vi "Dashboard Main.vi"() -> ()   [LabVIEW 2014]
uses:
  Autonomous Type.ctl
  <vilib>/event_ctls.llb/eventvkey.ctl
  <vilib>/Rock Robotics/WPI/Dashboard/WPI_DashboardLogging Global.vi
  <vilib>/Rock Robotics/Network Tables/SD Write Number.vi
  <vilib>/Rock Robotics/Network Tables/SD Read Number.vi
  <vilib>/Utility/config.llb/Write Key (String).vi
  <vilib>/Utility/config.llb/Write Key (I32).vi
  <vilib>/Utility/config.llb/NI_LVConfig.lvlib
panel:
  in  "TCP":refnum<k5>
  in  "Rec Mode":enum32{"Stop", "Record", "Playback"}(radio)
  in  "Vision":u16(ring) items=["Camera Off", "USB Camera SW", "USB Camera HW", "IP Camera"]
  out "Camera IP":string
  out "Image Message":string="Timeout in Camera Communications"
  in  "Dashboard Tab":T1(tab)
  out "Atonomous Type By Charlie":string
  in  "Camera Settings":T2={"Frame Rate"=30, "Compression"=30, "Size"=1} {"Frame Rate" scale=1.0..30.0; "Size" items=["640x480", "320x240", "160x120"]}
  out "MotorChart R":cluster{"Numeric":dbl, "Numeric":dbl}(graph)
  out "MotorChart L":T3(graph)
  out "MotorSliders R":cluster{"MotorSlide1":dbl, "MotorSlide2":dbl} {"MotorSlide2" scale=-1.0..1.0 scale format="%#_2e"; "MotorSlide1" scale=-1.0..1.0 scale format="%#_2e"}
  out "MotorSliders L":T4 {"MotorSlide4 2" scale=0.0..14.0 scale format="%#_2e"; "MotorSlide2" scale=-1.0..1.0 scale format="%#_2e"; "MotorSlide1" scale=-1.0..1.0 scale format="%#_2e"}
  out "Gyro":dbl(knob) scale=0.0..360.0
  out "JS1 Z":dbl(slide) scale=-1.0..1.0 scale format="%#_2e"
  out "JS1 Graph":cluster{"X":dbl, "Y":dbl}[](graph)
  out "JS1 Buttons":T5
  out "JS2 Z":dbl(slide) scale=-1.0..1.0 scale format="%#_2e"
  out "JS2 Graph":cluster{"X":dbl, "Y":dbl}[](graph)
  out "JS2 Buttons":T5
  out "Mode":T6(ring)=enum."Auto Disabled"
  in  "DB Camera Config":bool
  out "fps":dbl format="%#.1g"
  out "Mbps":dbl format="%#.1g"
  out "Mbps 2":bool
  in  "DB/String 9":string
  in  "DB/String 8":string
  in  "DB/String 7":string
  in  "DB/String 6":string
  in  "DB/String 5":string
  in  "DB/String 4":string
  in  "DB/String 3":string
  in  "DB/String 2":string
  in  "DB/String 1":string
  in  "DB/String 0":string
  in  "DB/Slider 0":dbl(slide) scale=0.0..5.0
  in  "DB/Slider 1":dbl(slide) scale=0.0..5.0
  in  "DB/Slider 2":dbl(slide) scale=0.0..5.0
  in  "DB/Slider 3":dbl(slide) scale=0.0..5.0
  out "DB/LED 3":bool
  out "DB/LED 2":bool
  out "DB/LED 1":bool
  out "DB/LED 0":bool
  in  "DB/Button 3":bool
  in  "DB/Button 2":bool
  in  "DB/Button 1":bool
  in  "DB/Button 0":bool caption="New Name"
  in  "Auto Type":T7
  in  "Test Slider":dbl(slide) scale=0.0..100.0 scale format="%#_3g"
  in  "On/Off":bool caption="Solenoid"
  in  "Test Name":u16(ring) items=["Select the test to run...", "Example Test", "-------------------------------", "List of tests is built in robot code.", "Replace with your own automated tests."]
  in  "Test Tree":string(tree)
  in  "Motor":cluster{"Value":dbl, "Enable":bool} {"Value" scale=-1.0..1.0 scale format="%#_3g"}
  out "Progress":T8 {"Test Progress" scale=0.0..100.0}
  in  "Rev/Fwd":cluster{"Forward":bool, "Reverse":bool}
  in  "Test Ring":u16(ring) items=["Monochrome", "Color"]
  in  "Listbox":i32(listbox)
  out "Tree":string(tree)
  out "Camera Image":T9(plugin-control)
  out "Boolean":bool
  # "Left"
  # "Front"
  # "Right"
  # "Battery"
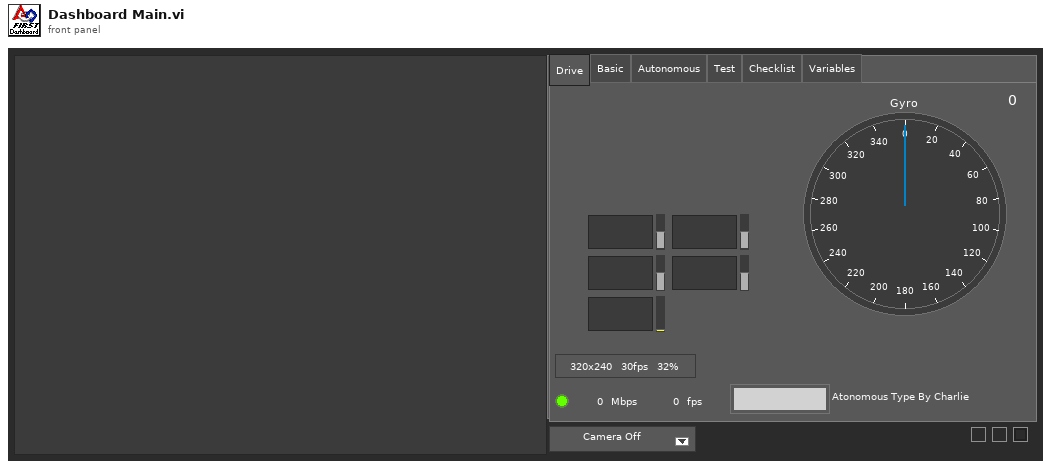
[diagram p1: front panel]
types:
  T1 = enum32{"Drive", "Basic", "Autonomous", "Test", "Checklist", "Variables"}
  T2 = cluster{"Frame Rate":i32, "Compression":i32, "Size":u16}
  T3 = cluster{"Numeric":dbl, "Numeric":dbl, "Battery V":dbl}
  T4 = cluster{"MotorSlide1":dbl, "MotorSlide2":dbl, "MotorSlide4 2":dbl}
  T5 = cluster{bool, bool, bool, bool, bool, bool, bool, bool, bool, bool, bool, bool}
  T6 = enum8{"Tele-Op Disabled", "Tele-Op Enabled", "Auto Disabled", "Auto Enabled", "Test Disabled", "Test Enabled", "Disconnected", "No Code", "E-Stop"}
  T7 = typedef "Autonomous Type.ctl" = enum16{"2 Totes + Turn", "Nothing", "3 Totes + Turn", "3 Totes + Strafe", "2 Totes + Strafe", "1 Tote", "Forward"}
  T8 = cluster{"Test Progress":u8, "Test Progress Text":string}
  T9 = typedef "IMAQ Image.ctl" = refnum<image>
  T10 = enum32{"Drive", "Basic", "Custom", "Test", "Checklist", "Variables"}
  T11 = typedef "Image Type" = u32
  T12 = cluster{"Camera Image":refnum<vi>, "Dashboard Tab":refnum<vi>, "Boolean":refnum<vi>, "Vision":refnum<vi>, "Rec Mode":refnum<vi>, "Test Slider":refnum<vi>, "On/Off ":refnum<vi>, "Test Ring":refnum<vi>, "Rev/Fwd":refnum<vi>, "Test Name":refnum<vi>, "Motor":refnum<vi>, "Progress":refnum<vi>, "CheckList":refnum<vi>, "Tree":refnum<vi>, "Test Tree":refnum<vi>}
  T13 = cluster{"Error Strings":string, "Disable Counts":cluster{u16, u16}, "Rail Faults":cluster{u16, u16, u16}, "Robot IP":string, "DB Mode":u8, "Event Info":cluster{"Name":string, "Type":u8, "Number":u16, "Replay":u8}, "Camera Addr":string}
  T14 = cluster{"Storage":cluster{"Disk Free":u64, "RAM Block":u32, "RAM free":u32}, "CPU Utilization":cluster{"CPU % ISR":sgl, "CPU % Time Crit":sgl, "CPU % Timed Str":sgl, "CPU % High":sgl, "CPU % Above":sgl, "CPU % Normal":sgl, "CPU % Low":sgl}, "CAN":cluster{"% Bus Utilization":sgl, "Bus Off Cnt":u32, "TX_FIFO Full Cnt":u32, "Receive Error Cnt":u8, "Transmit Error Cnt":u8}, "HID":cluster{"HID Outputs":u32, "Rumble Low":u16, "Rumble High":u16}[]}
  T15 = cluster{"Status bits":cluster{"Test Mode":bool, "Autonomous":bool, "Enabled":bool, "Code Start":bool, "Brownout":bool, "Reserved 2":bool, "Reserved 3":bool, "E-Stop":bool}, "Code Trace":cluster{"Disabled":bool, "TeleOp":bool, "Auto":bool, "Test":bool}, "Controller Type":enum16{"unknown", "cRIO", "roboRio"}, "Code?":enum16{"unknown", "noCode", "code"}, "Battery V":dbl}
  T16 = cluster{"Control Bits":cluster{"TestMode":bool, "Autonomous":bool, "Enabled":bool, "FMS Present":bool, bool, bool, bool, "E-Stop":bool}, "Team Station ":u8, "Countdown":sgl, "Joystick Values":cluster{"Axes":dbl[], "Buttons":bool[], "POVs":i16[]}[]}
  T17 = cluster{"Axes":dbl[], "Buttons":bool[], "POVs":i16[]}[]
  T18 = cluster{"Axes":dbl[], "Buttons":bool[], "POVs":i16[]}
  T19 = cluster{"Buttons[0]":bool, "Buttons[1]":bool, "Buttons[2]":bool, "Buttons[3]":bool, "Buttons[4]":bool, "Buttons[5]":bool, "Buttons[6]":bool, "Buttons[7]":bool, "Buttons[8]":bool, "Buttons[9]":bool, "Buttons[10]":bool, "Buttons[11]":bool}
  T20 = typedef "NI_LVConfig.lvlib/Config Data RefNum.ctl" = refnum<k1>
  T21 = cluster{"Operation":enum16{"Update", "Clear"}, "Color Box":u32}[]
  T22 = typedef "eventvkey.ctl" = enum16{"ASCII", "Enter", "Return", "Shift", "Ctrl", "Alt", "Cmd", "Opt", "Caps", "NumLock", "Clear", "Break", "Up", "Down", "Left", "Right", "Insert", "Delete", "Home", "End", "PageUp", "PageDown", "Escape", "Help", "Pause", "ScrollLock", "F1", "F2", "F3", "F4", "F5", "F6", "F7", "F8", "F9", "F10", "F11", "F12", "F13", "F14", "F15", "F16", "F17", "F18", "F19", "F20", "F21", "F22", "F23", "F24", "Play", "VolumeUp", "VolumeDown", "Mute", "Two Byte Char"}
  T23 = cluster{"Image Size":bool, "Image Type":bool, "Pixel Value":bool, "ROI Information":bool, "Zoom Factor":bool}
  T24 = enum8{"Enabled", "Disabled", "Disabled and Grayed Out"}
  T25 = cluster{"Operation":enum16{"Update", "Clear"}, "Color Box":u32}
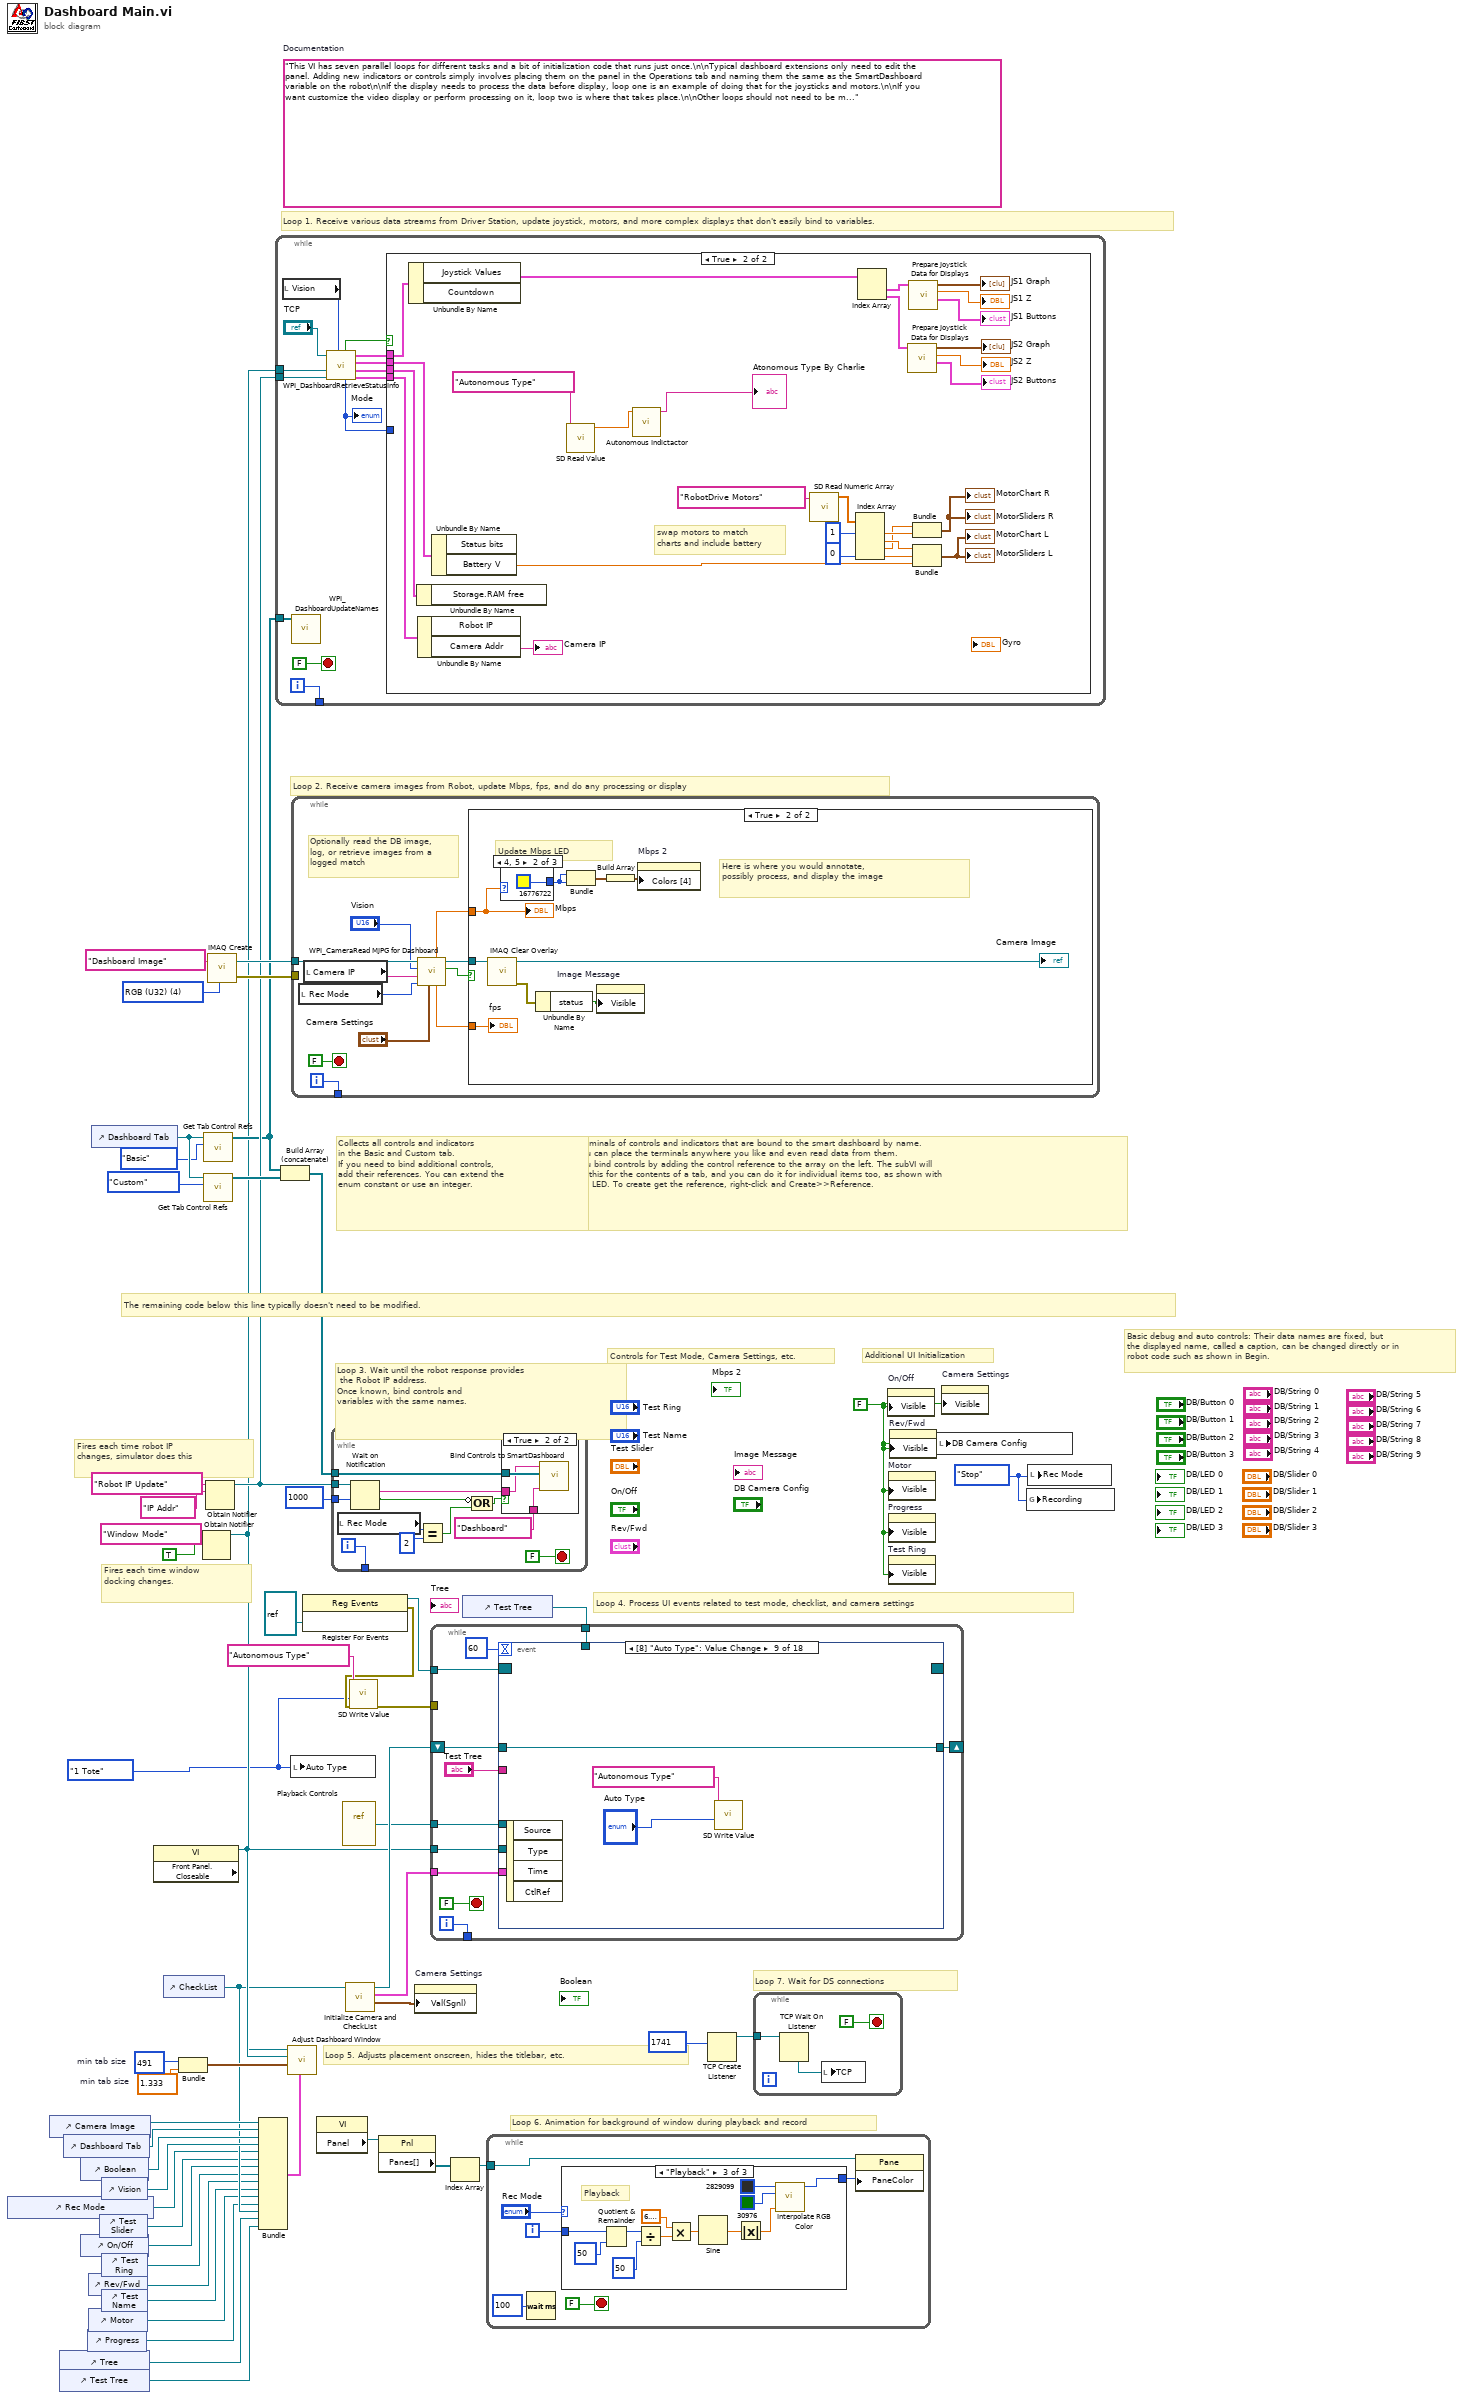
[diagram p0: block diagram]
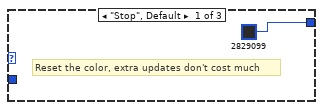
[diagram p3: hidden frame]
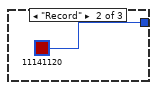
[diagram p4: hidden frame]
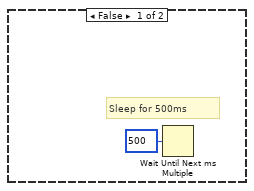
[diagram p6: hidden frame]
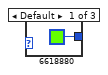
[diagram p7: hidden frame]
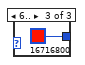
[diagram p8: hidden frame]
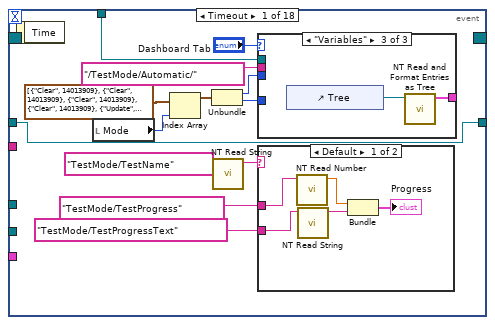
[diagram p9: hidden frame]
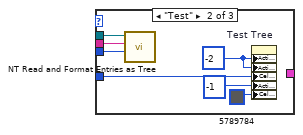
[diagram p11: hidden frame]
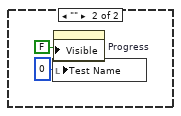
[diagram p12: hidden frame]
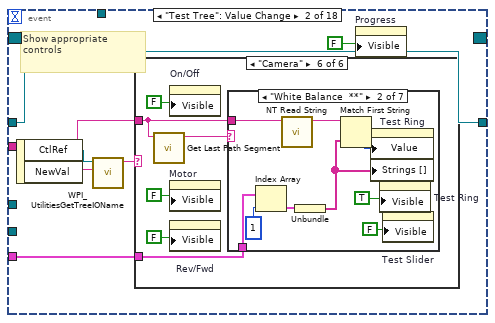
[diagram p13: hidden frame]
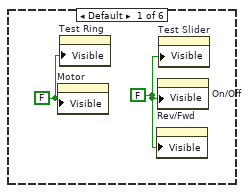
[diagram p14: hidden frame]
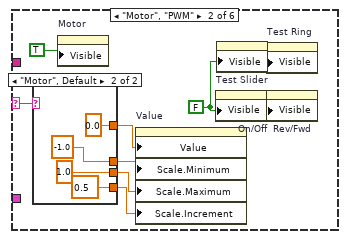
[diagram p15: hidden frame]
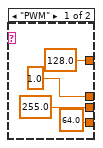
[diagram p16: hidden frame]
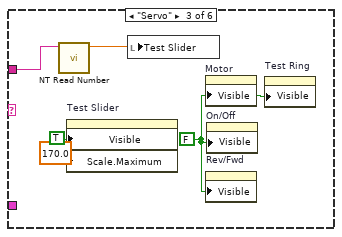
[diagram p17: hidden frame]
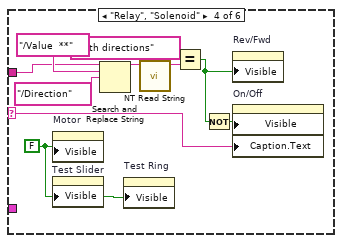
[diagram p18: hidden frame]
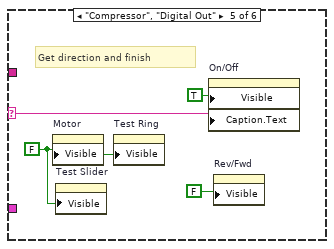
[diagram p19: hidden frame]
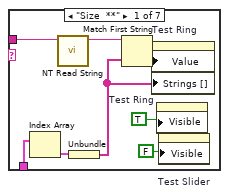
[diagram p20: hidden frame]
diagram:
  w1 = Autonomous_Type."1 Tote" ("Auto Type")
  w28 = 491  # min tab size
  w27 = 1.333  # min tab size
  w36 = enum32{"Stop", "Record", "Playback"}."Stop" ("Rec Mode")
  w10 = FALSE ("Visible")
  (unwired) "This VI has seven parallel loops for different tasks and a bit of initialization code that runs just once.\n\nTypical dashboard extensions only need to edit the panel. Adding new indicators or controls simply involves placing them on the panel in the Operations tab and naming them the same as the SmartDashboard variable on the robot\n\nIf the display needs to process the data before display, loop one is an example of doing that for the joysticks and motors.\n\nIf you want customize the video display or perform processing on it, loop two is where that takes place.\n\nOther loops should not need to be modified. They are pretty standard, and document the task they perform."  # Documentation
  w55 = T11 4 items=["Grayscale (U8)", "Grayscale (I16)", "Grayscale (SGL)", "Complex (CSG)", "RGB (U32)", "HSL (U32)", "RGB (U64)"] ("Image Type")
  # "Loop 7. Wait for DS connections"
  # "Basic debug and auto controls: Their data names are fixed, but\nthe displayed name, called a caption, can be changed directly or in\nrobot code such as shown in Begin."
  # "Controls for Test Mode, Camera Settings, etc."
  # "Additional UI Initialization"
  # "Loop 6. Animation for background of window during playback and record"
  # "Fires each time robot IP\nchanges, simulator does this"
  # "Fires each time window\ndocking changes."
  # "Collects all controls and indicators\nin the Basic and Custom tab.\nIf you need to bind additional controls,\nadd their references. You can extend the\nenum constant or use an integer."
  # "The remaining code below this line typically doesn't need to be modified."
  # "Loop 4. Process UI events related to test mode, checklist, and camera settings"
  # "Terminals of controls and indicators that are bound to the smart dashboard by name.\nYou can place the terminals anywhere you like and even read data from them.\nYou bind controls by adding the control reference to the array on the left. The subVI will\ndo this for the contents of a tab, and you can do it for individual items too, as shown with\nthe LED. To create get the reference, right-click and Create>>Reference."
  # "Loop 3. Wait until the robot response provides\n the Robot IP address.\nOnce known, bind controls and\nvariables with the same names."
  # "Loop 5. Adjusts placement onscreen, hides the titlebar, etc."
  # "Loop 1. Receive various data streams from Driver Station, update joystick, motors, and more complex displays that don't easily bind to variables."
  # "Loop 2. Receive camera images from Robot, update Mbps, fps, and do any processing or display"
  n1 = control-ref of="Rec Mode"() -> (w16:refnum<vi>)
  n2 = control-ref of="Camera Image"() -> (w31:refnum<vi>)
  n3 = control-ref of="Tree"() -> (w20:refnum<vi>)
  n4 = control-ref of="Test Tree"() -> (w19:refnum<vi>)
  n5 = control-ref of="Dashboard Tab"() -> (w30:refnum<vi>)
  n6 = control-ref of="Boolean"() -> (w25:refnum<vi>)
  n7 = control-ref of="On/Off"() -> (w14:refnum<vi>)
  n8 = control-ref of="Progress"() -> (w11:refnum<vi>)
  n9 = control-ref of="Rev/Fwd"() -> (w12:refnum<vi>)
  n10 = control-ref of="Motor"() -> (w17:refnum<vi>)
  n11 = control-ref of="Dashboard Tab"() -> (w34:refnum<vi>)
  n12 = control-ref of="Test Slider"() -> (w15:refnum<vi>)
  n13 = control-ref of="Vision"() -> (w29:refnum<vi>)
  n14 = control-ref of="Test Ring"() -> (w13:refnum<vi>)
  n15 = control-ref of="Test Name"() -> (w18:refnum<vi>)
  n16 = property class="VI" props=["Front Panel.Closeable"]() -> (reference out=w35:refnum<vi>)  [unwired: 2 in, 2 out]
  n17 = control-ref of="CheckList"() -> (w21:refnum<vi>)
  n18 = Bundle("min tab size"=w28, "min tab size"=w27) -> (w26:cluster{"min tab size":i32, "min tab size":dbl})  [unwired: 1 in]
  n19 = Obtain Notifier(name (unnamed)="Window Mode", notification data type=TRUE) -> (notifier out=w7:refnum<notifier>)  [unwired: 2 in, 2 out]
  n20 = call <vilib>:"Get Tab Control Refs.vi"("Page Index"=T10."Basic" ("Dashboard Tab"), "TabControl in"=w34) -> ("ControlsOnPage"=w8:refnum<vi>[])  [unwired: 9 in]
  n21 = call <vilib>:"Get Tab Control Refs.vi"("Page Index"=T10."Custom" ("Dashboard Tab"), "TabControl in"=w34) -> ("ControlsOnPage"=w33:refnum<vi>[])  [unwired: 9 in]
  n22 = Obtain Notifier(name (unnamed)="Robot IP Update", notification data type="IP Addr" ("name (unnamed)")) -> (notifier out=w9:refnum<notifier>)  [unwired: 2 in, 2 out]
  n23 = call "IMAQ Create"("Image Name"="Dashboard Image", "Image Type"=w55) -> ("New Image"=w53:T9, "error out"=w52:errorcluster)  [unwired: 2 in, 1 out]
  n24 = Bundle("Camera Image"=w31, "Dashboard Tab"=w30, "Boolean"=w25, "Vision"=w29, "Rec Mode"=w16, "Test Slider"=w15, "On/Off"=w14, "Test Ring"=w13, "Rev/Fwd"=w12, "Test Name"=w18, "Motor"=w17, "Progress"=w11, "CheckList"=w21, "Tree"=w20, "Test Tree"=w19) -> (w22:T12)  [unwired: 1 in]
  n25 = while {
    tunnel: [w67] -> _
    tunnel: w9 -> [w61]
    tunnel: w8 -> [w60]
    tunnel: w7 -> [w56]
    i -> [w67]
    stop <- FALSE stop-if-true
    n26 = local read "Vision"() -> (w58:u16)
    n27 = call <vilib>:"WPI_DashboardUpdateNames.vi"("Controls on Tab"=w60) -> ()  [unwired: 11 in]
    n28 = call <vilib>:"WPI_DashboardRetrieveStatusInfo.vi"("Vision"=w58, "Binding Refnum"=w61, "Window Mode Notifier"=w56, "TCP Cnx"="TCP") -> ("Power and Errors"=w62:T13, "Robot Metrics"=w65:T14, "Status Info"=w66:T15, "Control Info"=w63:T16, "Robot Mode"=w59:T6, "Process?"=w64:bool)  [unwired: 2 in]
    "Mode" <- w59
    n29 = case shown="True" w64 {
      tunnel: w66 -> [_ w96]
      tunnel: w65 -> [_ w95]
      tunnel: w63 -> [_ w94]
      tunnel: w62 -> [_ w93]
      tunnel: w59 -> [_ _]
      frame False {
      }
      frame True {
        # "swap motors to match\ncharts and include battery"
        n30 = Unbundle By Name(w94) -> ("Joystick Values"=w81:T17)  [unwired: 1 out]
        n31 = Unbundle By Name(w95) -> ()  [unwired: 1 out]
        n32 = Unbundle By Name(w93) -> ("Camera Addr"=→"Camera IP":string)  [unwired: 1 out]
        n33 = Unbundle By Name(w96) -> ("Battery V"=w82:dbl)  [unwired: 1 out]
        n34 = call-poly <vilib>:"SD Read Value.vi"("Name"="Autonomous Type") -> ("Numeric"=w70:dbl)  [unwired: 8 in, 2 out]
        n35 = call "Autonomous Indictactor.vi"("Int In"=w70) -> ("String Out"=→"Atonomous Type By Charlie":string)  [unwired: 10 in]
        n36 = call <vilib>:"SD Read Numeric Array.vi"("Name"="RobotDrive Motors") -> ("Numeric Array"=w84:dbl[])  [unwired: 8 in, 2 out]
        n37 = Index Array(array=w84, index #1=1, index #4=0) -> (element #1=w88:dbl, element #2=w89:dbl, element #3=w87:dbl, element #4=w92:dbl)  [unwired: 2 in]
        n38 = Index Array(array=w81) -> (element #1=w80:T18, element #2=w75:T18)  [unwired: 2 in]
        n39 = call "Prepare Joystick Data for Displays.vi"("Joystick Values"=w75) -> ("Buttons"=→"JS2 Buttons":T19, "Z Axis"=→"JS2 Z":dbl, "Cartesian Data"=→"JS2 Graph":cluster{"X axis":dbl, "X axis":dbl}[])  [unwired: 8 in]
        n40 = call "Prepare Joystick Data for Displays.vi"("Joystick Values"=w80) -> ("Buttons"=→"JS1 Buttons":T19, "Z Axis"=→"JS1 Z":dbl, "Cartesian Data"=→"JS1 Graph":cluster{"X axis":dbl, "X axis":dbl}[])  [unwired: 8 in]
        n41 = Bundle("Numeric"=w87, "Numeric"=w88) -> (→"MotorChart R" →"MotorSliders R":cluster{"Numeric":dbl, "Numeric":dbl})  [unwired: 1 in]
        n42 = Bundle("Numeric"=w89, "Numeric"=w92, "Battery V"=w82) -> (→"MotorChart L" →"MotorSliders L":T3)  [unwired: 1 in]
      }
    }
  }
  n43 = Build Array (concatenate)(w8, w33) -> (w32:refnum<vi>[])
  n44 = call "Adjust Dashboard Window.vi"("Sizing Refnums"=w22, "Size Constraints"=w26, "VI"=w35, "Notifier in"=w7) -> ()  [unwired: 8 in]
  n45 = local write "Auto Type"(w1) -> ()
  n46 = while {
    tunnel: w53 -> [w105]
    tunnel: w52 -> [_]
    tunnel: [w106] -> _
    i -> [w106]
    stop <- FALSE stop-if-true
    # "Optionally read the DB image,\nlog, or retrieve images from a\nlogged match"
    n47 = local read "Rec Mode"() -> (w99:enum32{"Stop", "Record", "Playback"})
    n48 = local read "Camera IP"() -> (w97:string)
    n49 = call <vilib>:"WPI_CameraRead MJPG for Dashboard.vi"("Camera Settings"="Camera Settings", "Rec Mode"=w99, "Camera IP"=w97, "Camera Mode"="Vision", "Refnum in"=w105) -> ("Active"=w103:bool, "Refnum out"=w104:T9, "FPS"=w102:dbl, "Bandwidth (Mbps)"=w101:dbl)  [unwired: 3 in]
    n50 = case shown="True" w103 {
      tunnel: w104 -> [_ w112]
      tunnel: w101 -> [_ w111]
      tunnel: w102 -> [_ w109]
      frame False {
        # "Sleep for 500ms"
        n51 = Wait Until Next ms Multiple(millisecond multiple=u32 500) -> ()  [unwired: 1 out]
      }
      frame True {
        # "Here is where you would annotate,\npossibly process, and display the image"
        # "Update Mbps LED"
        n52 = call "IMAQ Clear Overlay"("Image"=w112) -> ("error out"=w116:errorcluster, "Image Out"=→"Camera Image":T9)  [unwired: 2 in, 7 out]
        n53 = case shown="4, 5" w111 {
          tunnel: [u32 6618880 ("Color Box") u32 16776722 ("Color Box") u32 16716800 ("Color Box")] -> w113
          frame Default {
          }
          frame 4, 5 {
          }
          frame 6.. {
          }
        }
        n54 = Unbundle By Name(w116) -> ("status"=w117:bool)
        n55 = Bundle("Color Box"=w113, "Color Box"=w113) -> (w115:cluster{"Color Box":u32, "Color Box":u32})  [unwired: 1 out]
        n56 = property on="Image Message" class="Str"("Visible"=w117) -> ()  [unwired: 2 in, 2 out]
        n57 = Build Array(w115) -> (w114:cluster{"Color Box":u32, "Color Box":u32}[])
        n58 = property on="Mbps 2" class="Bool (strict)"("Colors [4]"=w114) -> ()  [unwired: 2 in, 2 out]
        "Mbps" <- w111
        "fps" <- w109
      }
    }
  }
  n59 = register-events(refnum<vi> refnum) -> (reference out=w39:refnum<event-registration>, error out=w3:errorcluster)  [unwired: 2 in]
  n60 = property class="VI"() -> ("Panel"=w42:refnum<vi>)  [unwired: 2 in, 2 out]
  n61 = while {
    tunnel: w32 -> [w132]
    tunnel: w9 -> [w130]
    tunnel: [w128] -> _
    tunnel: u32 1000 ("milliseconds to wait") -> [w127]
    i -> [w128]
    stop <- FALSE stop-if-true
    n62 = local read "Rec Mode"() -> (w123:enum32{"Stop", "Record", "Playback"})
    n63 = Wait on Notification(notifier=w130, timeout in ms (-1)=w127) -> (notification=w129:string, timed out?=w125:bool)  [unwired: 2 in, 2 out]
    n64 = Equal?(x=w123, y=u16 2 ("Rec Mode")) -> (x = y?=w124:bool)
    n65 = Compound Arithmetic op=OR(invert w125, w124) -> (w126:bool)
    n66 = case shown="True" w126 {
      tunnel: w132 -> [_ w135]
      tunnel: w129 -> [_ w134]
      tunnel: "Dashboard" -> [_ w133]
      frame False {
      }
      frame True {
        n67 = call <vilib>:"Bind Controls to SmartDashboard.vi"("Client Name"=w133, "Bound Control Refs"=w135, "Server IP Address"=w134) -> ()  [unwired: 9 in]
      }
    }
  }
  n68 = vi-ref "Playback Controls.vi"() -> (w40:refnum<vi>)
  n69 = call "Initialize Camera and CheckList.vi"("ListBox in"=w21) -> ("Cluster"=w46:cluster{"value":i32, "value":i32, "index":i32}, "Array"=w47:cluster{string[]}[], "File Refnum"=w45:T20)  [unwired: 8 in]
  n70 = call-poly <vilib>:"SD Write Value.vi"("error in"=w3, "Numeric"=w1, "Name"="Autonomous Type") -> ("error out"=w2:errorcluster)  [unwired: 7 in, 1 out]
  n71 = property class="Pnl"(reference=w42) -> ("Panes[]"=w43:refnum<vi>[])  [unwired: 1 in, 2 out]
  n72 = property on="Camera Settings" class="Clust (strict)"("Val(Sgnl)"=w46) -> ()  [unwired: 2 in, 2 out]
  n73 = Index Array(array=w43) -> (element=w41:refnum<vi>)  [unwired: 1 in]
  n74 = control-ref of="Test Tree"() -> (w44:refnum<vi>)
  n75 = while {
    tunnel: w47 -> [w143]
    shift-right: [w142] -> _
    shift-left: w45 -> [w141]
    tunnel: [w140] -> _
    tunnel: w44 -> [w139]
    tunnel: w40 -> [w138]
    tunnel: w39 -> [w137]
    tunnel: w35 -> [w136]
    tunnel: w2 -> [_]
    i -> [w140]
    stop <- FALSE stop-if-true
    n76 = event shown="[8] \"Auto Type\": Value Change" {
      selector: w137 -> [_ _ _ _ _ _ _ _ _ _ _ _ _ _ _ _ _ _]
      dyn-events: [_ _ _ _ _ _ _ _ _ _ _ _ _ _ w384 _ _ _] -> _
      timeout: u32 60 ("milliseconds to wait") -> [_ _ _ _ _ _ _ _ _ _ _ _ _ _ _ _ _ _]
      tunnel: w139 -> [w155 _ _ _ _ _ _ _ _ _ _ _ _ _ _ _ _ _]
      tunnel: "Test Tree" -> [_ _ _ _ _ _ _ _ _ w353 w361 w363 w367 w375 _ _ _ _]
      tunnel: w143 -> [_ w177 _ _ _ _ w314 w344 _ _ _ _ _ _ _ _ _ _]
      tunnel: [w151 w176 w275 w280 w288 w300 w313 w337 w351 w352 w359 w362 w366 w374 w386 w400 w401 w411] -> w142
      tunnel: w141 -> [w151 w176 w275 w280 w288 w300 w312 w337 w351 w352 w359 w362 w366 w374 w386 w400 w401 w411]
      tunnel: w138 -> [_ _ _ _ _ _ _ _ _ _ _ _ _ _ w387 _ w404 _]
      tunnel: w136 -> [_ _ _ _ _ _ _ _ _ _ _ _ _ _ w382 _ _ _]
      event Timeout {
        n77 = event-data() -> ()  [unwired: 1 in, 1 out]
        n78 = local read "Mode"() -> (w154:T6)
        n79 = Index Array(array=T21 [{"Operation"=enum."Clear", "Color Box"=14013909}, {"Operation"=enum."Clear", "Color Box"=14013909}, {"Operation"=enum."Clear", "Color Box"=14013909}, {"Operation"=enum."Clear", "Color Box"=14013909}, {"Operation"=enum."Update", "Color Box"=14013909}, {"Operation"=enum."Update", "Color Box"=16777215}, {"Operation"=enum."Clear", "Color Box"=14013909}, {"Operation"=enum."Clear", "Color Box"=14013909}, {"Operation"=enum."Clear", "Color Box"=14013909}], index=w154) -> (element=w149:T25)
        n80 = Unbundle(w149) -> ("Operation"=w148:enum16{"Update", "Clear"}, "Color Box"=w147:u32)
        n81 = call <vilib>:"NT Read String.vi"("Name"="TestMode/TestName") -> ("String"=w158:string)  [unwired: 9 in, 1 out]
        n82 = case shown="\"Variables\"" "Dashboard Tab" {
          tunnel: w155 -> [_ w166 _]
          tunnel: "/TestMode/Automatic/" ("Name Pattern") -> [_ w165 _]
          tunnel: w148 -> [_ w164 _]
          tunnel: [_ _ w168] -> _
          tunnel: w147 -> [_ w160 _]
          frame "Autonomous", Default {
          }
          frame "Test" {
            w163 = -2 ("Active Item:Row Number")
            n83 = call <vilib>:"NT Read and Format Entries as Tree.vi"("Operation"=w164, "Name Pattern"=w165, "Tree Refnum"=w166) -> ()  [unwired: 7 in, 2 out]
            n84 = property on="Test Tree" class="Tree (strict)"("Active Item Row Number"=w163, "ActiveColNum"=w163, "CellBG"=w160, "Active Item Row Number"=-1 ("Active Item:Row Number"), "CellBG"=u32 5789784 ("Color Box")) -> ()  [unwired: 2 in, 2 out]
          }
          frame "Variables" {
            n85 = control-ref of="Tree"() -> (w167:refnum<vi>)
            n86 = call <vilib>:"NT Read and Format Entries as Tree.vi"("Tree Refnum"=w167) -> ("Formatted Strings"=w168:cluster{"Name":string, "Value":string}[])  [unwired: 9 in, 1 out]
          }
        }
        n87 = case shown="Default" w158 {
          tunnel: "TestMode/TestProgress" ("Name") -> [w170 _]
          tunnel: "TestMode/TestProgressText" ("Name") -> [w169 _]
          frame Default {
            n88 = call <vilib>:"NT Read Number.vi"("Name"=w170) -> ("Numeric"=w171:dbl)  [unwired: 9 in, 1 out]
            n89 = call <vilib>:"NT Read String.vi"("Name"=w169) -> ("String"=w172:string)  [unwired: 9 in, 1 out]
            n90 = Bundle("Numeric"=w171, "String"=w172) -> (→"Progress":cluster{"Numeric":dbl, "String":string})  [unwired: 1 in]
          }
          frame "" {
            n91 = local write "Test Name"(u16 0) -> ()
            n92 = property on="Progress" class="Clust (strict)"("Visible"=FALSE) -> ()  [unwired: 2 in, 2 out]
          }
        }
      }
      event "Test Tree": Value Change {
        # "Show appropriate\ncontrols"
        n93 = event-data() -> ("CtlRef"=w180:refnum<vi>, "NewVal"=w178:string)  [unwired: 1 in]
        n94 = call <vilib>:"WPI_UtilitiesGetTreeIOName.vi"("NewVal"=w178, "TreeControl in"=w180) -> ("I/O Name"=w181:string)  [unwired: 9 in]
        n95 = case shown="\"Camera\"" w181 {
          selector: w181 -> [_ w188 _ w206 w215 _]
          tunnel: w178 -> [_ _ w203 w205 _ w222]
          tunnel: w177 -> [_ _ _ _ _ w221]
          frame Default {
            w183 = FALSE ("Visible")
            w182 = FALSE ("Visible")
            n96 = property on="Motor" class="Clust (strict)"("Visible"=w182) -> ()  [unwired: 2 in, 2 out]
            n97 = property on="Test Ring" class="Ring (strict)"("Visible"=w182) -> ()  [unwired: 2 in, 2 out]
            n98 = property on="Rev/Fwd" class="Clust (strict)"("Visible"=w183) -> ()  [unwired: 2 in, 2 out]
            n99 = property on="On/Off" class="Bool (strict)"("Visible"=w183) -> ()  [unwired: 2 in, 2 out]
            n100 = property on="Test Slider" class="Slide (strict)"("Visible"=w183) -> ()  [unwired: 2 in, 2 out]
          }
          frame "Motor", "PWM" {
            w189 = FALSE ("Visible")
            n101 = case shown="\"Motor\", Default" w188 {
              tunnel: [1.0 ("Value") -1.0 ("Value")] -> w187
              tunnel: [255.0 ("Value") 1.0 ("Value")] -> w186
              tunnel: [128.0 ("Value") 0.0 ("Value")] -> w185
              tunnel: [64.0 ("Value") 0.5 ("Value")] -> w184
              frame "PWM" {
              }
              frame "Motor", Default {
              }
            }
            n102 = property on="Motor" class="Clust (strict)"("Visible"=TRUE) -> ()  [unwired: 2 in, 2 out]
            n103 = property on="Value" class="Slide (strict)"("Value"=w185, "Scale.Minimum"=w187, "Scale.Maximum"=w186, "Scale.Increment"=w184) -> ()  [unwired: 2 in, 2 out]
            n104 = property on="On/Off" class="Bool (strict)"("Visible"=w189) -> ()  [unwired: 2 in, 2 out]
            n105 = property on="Test Slider" class="Slide (strict)"("Visible"=w189) -> ()  [unwired: 2 in, 2 out]
            n106 = property on="Test Ring" class="Ring (strict)"("Visible"=w189) -> ()  [unwired: 2 in, 2 out]
            n107 = property on="Rev/Fwd" class="Clust (strict)"("Visible"=w189) -> ()  [unwired: 2 in, 2 out]
          }
          frame "Servo" {
            w201 = FALSE ("Visible")
            n108 = call <vilib>:"NT Read Number.vi"("Name"=w203) -> ("Numeric"=w202:dbl)  [unwired: 9 in, 1 out]
            n109 = property on="Test Slider" class="Slide (strict)"("Visible"=TRUE, "Scale.Maximum"=170.0 ("Scale.Range:Maximum")) -> ()  [unwired: 2 in, 2 out]
            n110 = local write "Test Slider"(w202) -> ()
            n111 = property on="Motor" class="Clust (strict)"("Visible"=w201) -> ()  [unwired: 2 in, 2 out]
            n112 = property on="Rev/Fwd" class="Clust (strict)"("Visible"=w201) -> ()  [unwired: 2 in, 2 out]
            n113 = property on="On/Off" class="Bool (strict)"("Visible"=w201) -> ()  [unwired: 2 in, 2 out]
            n114 = property on="Test Ring" class="Ring (strict)"("Visible"=w201) -> ()  [unwired: 2 in, 2 out]
          }
          frame "Relay", "Solenoid" {
            w204 = FALSE ("Visible")
            n115 = property on="Motor" class="Clust (strict)"("Visible"=w204) -> ()  [unwired: 2 in, 2 out]
            n116 = property on="Test Slider" class="Slide (strict)"("Visible"=w204) -> ()  [unwired: 2 in, 2 out]
            n117 = Search and Replace String(input string=w205, search string="/Value  **", replace string="/Direction") -> (result string=w211:string)  [unwired: 5 in, 3 out]
            n118 = property on="Test Ring" class="Ring (strict)"("Visible"=w204) -> ()  [unwired: 2 in, 2 out]
            n119 = call <vilib>:"NT Read String.vi"("Name"=w211) -> ("String"=w209:string)  [unwired: 9 in, 1 out]
            n120 = Equal?(x="Both directions", y=w209) -> (x = y?=w207:bool)
            n121 = Not(x=w207) -> (.not. x?=w208:bool)
            n122 = property on="Rev/Fwd" class="Clust (strict)"("Visible"=w207) -> ()  [unwired: 2 in, 2 out]
            n123 = property on="On/Off" class="Bool (strict)"("Visible"=w208, "Caption.Text"=w206) -> ()  [unwired: 2 in, 2 out]
          }
          frame "Compressor", "Digital Out" {
            w214 = FALSE ("Visible")
            # "Get direction and finish"
            n124 = property on="Motor" class="Clust (strict)"("Visible"=w214) -> ()  [unwired: 2 in, 2 out]
            n125 = property on="Test Slider" class="Slide (strict)"("Visible"=w214) -> ()  [unwired: 2 in, 2 out]
            n126 = property on="Test Ring" class="Ring (strict)"("Visible"=w214) -> ()  [unwired: 2 in, 2 out]
            n127 = property on="On/Off" class="Bool (strict)"("Visible"=TRUE, "Caption.Text"=w215) -> ()  [unwired: 2 in, 2 out]
            n128 = property on="Rev/Fwd" class="Clust (strict)"("Visible"=FALSE) -> ()  [unwired: 2 in, 2 out]
          }
          frame "Camera" {
            n129 = call <vilib>:"Get Last Path Segment.vi"("String in"=w222) -> ("String out"=w223:string)  [unwired: 10 in]
            n130 = property on="On/Off" class="Bool (strict)"("Visible"=FALSE) -> ()  [unwired: 2 in, 2 out]
            n131 = property on="Motor" class="Clust (strict)"("Visible"=FALSE) -> ()  [unwired: 2 in, 2 out]
            n132 = property on="Rev/Fwd" class="Clust (strict)"("Visible"=FALSE) -> ()  [unwired: 2 in, 2 out]
            n133 = case shown="\"White Balance  **\"" w223 {
              tunnel: w222 -> [w229 w238 w247 w256 w265 _ w271]
              tunnel: w221 -> [w227 w235 w244 w253 w262 _ _]
              frame "Size  **" {
                n134 = Index Array(array=w227) -> (element=w226:cluster{string[]})  [unwired: 1 in]
                n135 = call <vilib>:"NT Read String.vi"("Name"=w229) -> ("String"=w228:string)  [unwired: 9 in, 1 out]
                n136 = Unbundle(w226) -> (w224:string[])
                n137 = Match First String(2:w224, 3:w228) -> (0:w225:i32)  [unwired: 1 out]
                n138 = property on="Test Ring" class="Ring (strict)"("Value"=w225, "Strings []"=w224) -> ()  [unwired: 2 in, 2 out]
                n139 = property on="Test Ring" class="Ring (strict)"("Visible"=TRUE) -> ()  [unwired: 2 in, 2 out]
                n140 = property on="Test Slider" class="Slide (strict)"("Visible"=FALSE) -> ()  [unwired: 2 in, 2 out]
              }
              frame "White Balance  **" {
                n141 = Index Array(array=w235, index=1) -> (element=w236:cluster{string[]})
                n142 = call <vilib>:"NT Read String.vi"("Name"=w238) -> ("String"=w237:string)  [unwired: 9 in, 1 out]
                n143 = Unbundle(w236) -> (w233:string[])
                n144 = Match First String(2:w233, 3:w237) -> (0:w232:i32)  [unwired: 1 out]
                n145 = property on="Test Ring" class="Ring (strict)"("Value"=w232, "Strings []"=w233) -> ()  [unwired: 2 in, 2 out]
                n146 = property on="Test Ring" class="Ring (strict)"("Visible"=TRUE) -> ()  [unwired: 2 in, 2 out]
                n147 = property on="Test Slider" class="Slide (strict)"("Visible"=FALSE) -> ()  [unwired: 2 in, 2 out]
              }
              frame "Exposure  **" {
                n148 = Index Array(array=w244, index=2) -> (element=w245:cluster{string[]})
                n149 = call <vilib>:"NT Read String.vi"("Name"=w247) -> ("String"=w246:string)  [unwired: 9 in, 1 out]
                n150 = Unbundle(w245) -> (w241:string[])
                n151 = Match First String(2:w241, 3:w246) -> (0:w242:i32)  [unwired: 1 out]
                n152 = property on="Test Ring" class="Ring (strict)"("Value"=w242, "Strings []"=w241) -> ()  [unwired: 2 in, 2 out]
                n153 = property on="Test Ring" class="Ring (strict)"("Visible"=TRUE) -> ()  [unwired: 2 in, 2 out]
                n154 = property on="Test Slider" class="Slide (strict)"("Visible"=FALSE) -> ()  [unwired: 2 in, 2 out]
              }
              frame "Exposure Priority  **" {
                n155 = Index Array(array=w253, index=3) -> (element=w254:cluster{string[]})
                n156 = call <vilib>:"NT Read String.vi"("Name"=w256) -> ("String"=w255:string)  [unwired: 9 in, 1 out]
                n157 = Unbundle(w254) -> (w250:string[])
                n158 = Match First String(2:w250, 3:w255) -> (0:w251:i32)  [unwired: 1 out]
                n159 = property on="Test Ring" class="Ring (strict)"("Value"=w251, "Strings []"=w250) -> ()  [unwired: 2 in, 2 out]
                n160 = property on="Test Ring" class="Ring (strict)"("Visible"=TRUE) -> ()  [unwired: 2 in, 2 out]
                n161 = property on="Test Slider" class="Slide (strict)"("Visible"=FALSE) -> ()  [unwired: 2 in, 2 out]
              }
              frame "Color Enable  **" {
                n162 = Index Array(array=w262, index=4) -> (element=w263:cluster{string[]})
                n163 = call <vilib>:"NT Read String.vi"("Name"=w265) -> ("String"=w264:string)  [unwired: 9 in, 1 out]
                n164 = Unbundle(w263) -> (w259:string[])
                n165 = Match First String(2:w259, 3:w264) -> (0:w260:i32)  [unwired: 1 out]
                n166 = property on="Test Ring" class="Ring (strict)"("Value"=w260, "Strings []"=w259) -> ()  [unwired: 2 in, 2 out]
                n167 = property on="Test Ring" class="Ring (strict)"("Visible"=TRUE) -> ()  [unwired: 2 in, 2 out]
                n168 = property on="Test Slider" class="Slide (strict)"("Visible"=FALSE) -> ()  [unwired: 2 in, 2 out]
              }
              frame Default {
                n169 = property on="Test Ring" class="Ring (strict)"("Visible"=FALSE) -> ()  [unwired: 2 in, 2 out]
                n170 = property on="Test Slider" class="Slide (strict)"("Visible"=FALSE) -> ()  [unwired: 2 in, 2 out]
              }
              frame "Brightness  **", "Color Level  **", "Compression  **", "FPS  **", "Sharpness  **" {
                n171 = call <vilib>:"NT Read Number.vi"("Name"=w271) -> ("Numeric"=w270:dbl)  [unwired: 9 in, 1 out]
                n172 = local write "Test Slider"(w270) -> ()
                n173 = property on="Test Slider" class="Slide (strict)"("Visible"=TRUE, "Scale.Maximum"=100.0 ("Scale.Range:Maximum")) -> ()  [unwired: 2 in, 2 out]
                n174 = property on="Test Ring" class="Ring (strict)"("Visible"=FALSE) -> ()  [unwired: 2 in, 2 out]
              }
            }
          }
        }
        n175 = property on="Progress" class="Clust (strict)"("Visible"=FALSE) -> ()  [unwired: 2 in, 2 out]
      }
      event "Test Name": Mouse Enter {
        # "Populate the ring with the list of tests"
        n176 = event-data() -> ()  [unwired: 1 in, 1 out]
        n177 = call <vilib>:"NT Read String Array.vi"("Name"="TestMode/TestList") -> ("String Array"=w279:string[])  [unwired: 9 in, 1 out]
        n178 = Build Array (concatenate)("Select the test to run...", w279) -> (w278:string[])
        n179 = property on="Test Name" class="Ring (strict)"("Strings []"=w278) -> ()  [unwired: 2 in, 2 out]
      }
      event "Test Name": Value Change {
        w281 = FALSE ("Visible")
        # "Tell the robot the test name to run"
        n180 = event-data() -> ("NewVal"=w285:u16)  [unwired: 1 in]
        n181 = property on="Test Name" class="Ring (strict)"() -> ("Strings []"=w286:string[])  [unwired: 2 in, 2 out]
        n182 = local write "Progress"(T8 {"Test Progress"=0, "Test Progress Text"=""} ("Progress")) -> ()
        n183 = Index Array(array=w286, index=w285) -> (element=w284:string)
        n184 = call <vilib>:"NT Write String.vi"("String"=w284, "Name"="TestMode/TestName") -> ()  [unwired: 9 in, 1 out]
        n185 = property on="Progress" class="Clust (strict)"("Visible"=TRUE) -> ()  [unwired: 2 in, 2 out]
        n186 = property on="Motor" class="Clust (strict)"("Visible"=w281) -> ()  [unwired: 2 in, 2 out]
        n187 = property on="Test Slider" class="Slide (strict)"("Visible"=w281) -> ()  [unwired: 2 in, 2 out]
        n188 = property on="On/Off" class="Bool (strict)"("Visible"=w281) -> ()  [unwired: 2 in, 2 out]
        n189 = property on="Rev/Fwd" class="Clust (strict)"("Visible"=w281) -> ()  [unwired: 2 in, 2 out]
        n190 = property on="Test Ring" class="Ring (strict)"("Visible"=w281) -> ()  [unwired: 2 in, 2 out]
      }
      event "Listbox": Double Click {
        # "Shift clears all"
        # "Update symbols on the listbox"
        n191 = event-data() -> ("PlatMods.Shift"=w289:bool, "Row"=w291:i32)  [unwired: 1 in]
        n192 = case shown="True" w289 {
          tunnel: w291 -> [w295 _]
          tunnel: 1 -> [w294 _]
          frame False {
            n193 = property on="Listbox" class="LstBox (strict)"() -> ("Item Symbols"=w293:i32[])  [unwired: 2 in, 2 out]
            n194 = Replace Array Subset(array=w293, new element=w294, index=w295) -> (w292:i32[])
            n195 = property on="Listbox" class="LstBox (strict)"("Item Symbols"=w292) -> ()  [unwired: 2 in, 2 out]
          }
          frame True {
            w296 = 0 ("Top Row")
            n196 = property on="Listbox" class="LstBox (strict)"() -> ("Number of Rows"=w298:u32)  [unwired: 2 in, 2 out]
            n197 = Initialize Array(0, w298) -> (w297:i32[])
            n198 = property on="Listbox" class="LstBox (strict)"("Top Row"=w296, "Value"=w296, "Item Symbols"=w297) -> ()  [unwired: 2 in, 2 out]
          }
        }
      }
      event "Listbox": Key Down {
        # "Update symbols on the listbox\nLeft and right keys check and uncheck"
        n199 = event-data() -> ("VKey"=w302:T22)  [unwired: 1 in]
        n200 = case shown="\"Left\", \"Right\"" w302 {
          selector: w302 -> [w307 _]
          tunnel: eventvkey."Left" ("VKey") -> [w305 _]
          frame "Left", "Right" {
            n201 = Equal?(x=w305, y=w307) -> (x = y?=w306:bool)
            n202 = Select(t=0, s=w306, f=1) -> (s? t:f=w308:i32)
            n203 = property on="Listbox" class="LstBox (strict)"() -> ("Item Symbols"=w311:i32[])  [unwired: 2 in, 2 out]
            n204 = Replace Array Subset(array=w311, new element=w308, index="Listbox") -> (w310:i32[])
            n205 = property on="Listbox" class="LstBox (strict)"("Item Symbols"=w310) -> ()  [unwired: 2 in, 2 out]
          }
          frame Default {
          }
        }
      }
      event "DB Camera Config": Value Change {
        # "Show or hide the cluster of controls, store in ini file"
        n206 = event-data() -> ("NewVal"=w315:bool)  [unwired: 1 in]
        n207 = case shown="False" w315 {
          tunnel: w314 -> [w324 _]
          tunnel: [w317 w335] -> w313
          tunnel: w312 -> [w316 w335]
          frame False {
            w331 = "Camera"
            w334 = FALSE ("Visible")
            n208 = local read "Camera Settings"() -> (w323:T2)
            n209 = Index Array(array=w324) -> (element=w327:cluster{string[]})  [unwired: 1 in]
            n210 = Unbundle(w323) -> ("Frame Rate"=w322:i32, "Compression"=w321:i32, "Size"=w325:u16)
            n211 = Unbundle(w327) -> (w326:string[])
            n212 = Index Array(array=w326, index=w325) -> (element=w320:string)
            n213 = call-poly <vilib>:"Write Key.vi"("section"=w331, "value"=w320, "key"="Size", "refnum"=w316) -> ("refnum out"=w333:T20)  [unwired: 2 in, 5 out]
            n214 = call-poly <vilib>:"Write Key.vi"("section"=w331, "value"=w322, "key"="FrameRate", "refnum"=w333) -> ("refnum out"=w332:T20)  [unwired: 1 in, 6 out]
            n215 = local write "DB Camera Config"(w334) -> ()
            n216 = property on="Camera Settings" class="Clust (strict)"("Visible"=w334) -> ()  [unwired: 2 in, 2 out]
            n217 = call-poly <vilib>:"Write Key.vi"("section"=w331, "value"=w321, "key"="Compression", "refnum"=w332) -> ("refnum out"=w318:T20)  [unwired: 1 in, 6 out]
            n218 = call <vilib>:"Close Config Data.vi"("refnum"=w318) -> ("file path"=w319:path)  [unwired: 2 in, 8 out]
            n219 = call <vilib>:"Open Config Data.vi"("configuration file path"=w319) -> ("refnum"=w317:T20)  [unwired: 8 in, 2 out]
          }
          frame True {
            n220 = property on="Camera Settings" class="Clust (strict)"("Visible"=TRUE) -> ()  [unwired: 2 in, 2 out]
          }
        }
      }
      event "Camera Settings": Value Change {
        # "Update summary string when any elements of DB camera change"
        n221 = event-data() -> ("NewVal"=w348:T2)  [unwired: 1 in]
        n222 = Index Array(array=w344) -> (element=w343:cluster{string[]})  [unwired: 1 in]
        n223 = Unbundle(w348) -> ("Frame Rate"=w339:i32, "Compression"=w338:i32, "Size"=w341:u16)
        n224 = Unbundle(w343) -> (w342:string[])
        n225 = Index Array(array=w342, index=w341) -> (element=w340:string)
        n226 = Format Into String(format string="%s   %dfps   %d%%", w340, w339, w338) -> (resulting string=w345:string)  [unwired: 2 in, 1 out]
        n227 = Build Array(w345) -> (w346:string[])
        n228 = property on="DB Camera Config" class="Bool (strict)"("Strings [4]"=w346) -> ()  [unwired: 2 in, 2 out]
      }
      event Value Change {
        n229 = event-data() -> ()  [unwired: 1 in, 4 out]
        n230 = call-poly <vilib>:"SD Write Value.vi"("Numeric"="Auto Type", "Name"="Autonomous Type") -> ()  [unwired: 8 in, 2 out]
      }
      event "Motor.Enable": Value Change {
        # "When the test mode otor enable helper is set, update that\ntree row item's value"
        n231 = event-data() -> ("NewVal"=w357:bool)  [unwired: 1 in]
        n232 = Unbundle("Motor") -> ("Value"=w356:dbl)  [unwired: 1 out]
        n233 = Select(t=w356, s=w357, f=0.0) -> (s? t:f=w354:dbl)
        n234 = call <vilib>:"NT Write Number.vi"("Numeric"=w354, "Name"=w353) -> ()  [unwired: 9 in, 1 out]
      }
      event "Test Slider": Value Change {
        # "When the test mode slider helper is set, update that\ntree row item's value"
        n235 = event-data() -> ("NewVal"=w360:dbl)  [unwired: 1 in]
        n236 = call <vilib>:"NT Write Number.vi"("Numeric"=w360, "Name"=w361) -> ()  [unwired: 9 in, 1 out]
      }
      event "On/Off": Value Change {
        # "When the test mode on/off helper value is set, update that\ntree row item's value"
        n237 = event-data() -> ("NewVal"=w365:bool)  [unwired: 1 in]
        n238 = Boolean To (0,1)(Boolean=w365) -> (0, 1=w364:i16)
        n239 = call <vilib>:"NT Write Number.vi"("Numeric"=w364, "Name"=w363) -> ()  [unwired: 9 in, 1 out]
      }
      event "Rev/Fwd": Value Change {
        # "When the test mode helper value for relays is set, update that\ntree row item's value"
        n240 = event-data() -> ("NewVal.Forward"=w373:bool, "NewVal.Reverse"=w372:bool)  [unwired: 1 in]
        n241 = Boolean To (0,1)(Boolean=w373) -> (0, 1=w369:i16)
        n242 = Boolean To (0,1)(Boolean=w372) -> (0, 1=w371:i16)
        n243 = Negate(x=w371) -> (-x=w370:i16)
        n244 = Add(x=w369, y=w370) -> (x+y=w368:i16)
        n245 = call <vilib>:"NT Write Number.vi"("Numeric"=w368, "Name"=w367) -> ()  [unwired: 9 in, 1 out]
      }
      event "Test Ring": Value Change {
        # "When a test mode helper value is selected from the ring,\nset the tree item's variable to the string value"
        n246 = event-data() -> ("NewVal"=w377:u16)  [unwired: 1 in]
        n247 = property on="Test Ring" class="Ring (strict)"() -> ("Strings []"=w378:string[])  [unwired: 2 in, 2 out]
        n248 = Index Array(array=w378, index=w377) -> (element=w376:string)
        n249 = call <vilib>:"NT Write String.vi"("String"=w376, "Name"=w375) -> ()  [unwired: 9 in, 1 out]
      }
      event "Rec Mode": Value Change {
        # "Update globals for recording mode and path to read log from.\nClear when logging and let NetworkTables set path for vision to\nuse."
        n250 = event-data() -> ("NewVal"=w388:enum32{"Stop", "Record", "Playback"})  [unwired: 1 in]
        n251 = global write "WPI_DashboardLogging Global.vi" "Logging Filename"(path "") -> ()
        n252 = global write "WPI_DashboardLogging Global.vi" "Recording"(w388) -> ()
        n253 = case shown="\"Playback\"" w388 {
          tunnel: w387 -> [_ w390 w398]
          tunnel: [_ _ w397] -> w384
          tunnel: [_ _ w396] -> _
          tunnel: w382 -> [_ _ w394]
          tunnel: cluster{i32, i32} {-250, 170} -> [_ _ w393]
          tunnel: [_ _ T23 {"Image Size"=TRUE, "Image Type"=TRUE, "Pixel Value"=TRUE, "ROI Information"=TRUE, "Zoom Factor"=FALSE} ("Image Information Shown:All Elements")] -> w380
          tunnel: [_ _ TRUE ("Zoom Factor")] -> w379
          frame Default {
          }
          frame "Stop", "Record" {
            # "Place Window too"
            n254 = invoke class="VI" method="FP.Close"(reference=w390) -> (reference out=w389:refnum<vi>)  [unwired: 2 in, 2 out]
            n255 = invoke class="VI" method="Abort VI"(reference=w389) -> ()  [unwired: 2 in, 3 out]
          }
          frame "Playback" {
            n256 = call "Open Playback Panel.vi"("Offset"=w393, "DB VI Ref"=w394, "Playback in"=w398) -> ("Playback out"=w395:refnum<vi>)  [unwired: 8 in]
            n257 = register-events(w395) -> (reference out=w397:refnum<event-registration>, error out=w396:errorcluster)  [unwired: 2 in]
          }
        }
        n258 = property on="Camera Image" class="ImageControl"("Image Information Shown"=w380, "Image Information Visible"=w379) -> ()  [unwired: 2 in, 2 out]
        n259 = call <vilib>:"WPI_DashboardNT Log FieldName Cache.vi"("Operation"=enum16{"Lookup/Add", "Index", "Clear"}."Clear") -> ()  [unwired: 8 in, 3 out]
      }
      event Panel Close {
        w399 = enum32{"Stop", "Record", "Playback"}."Stop" ("Rec Mode")
        # "Playback window has been closed, abort"
        n260 = event-data() -> ()  [unwired: 1 in, 4 out]
        n261 = local write "Rec Mode"(w399) -> ()
        n262 = global write "WPI_DashboardLogging Global.vi" "Recording"(w399) -> ()
      }
      event Panel Close {
        # "Abort playback window and ourself"
        n263 = event-data() -> ()  [unwired: 1 in, 4 out]
        n264 = invoke class="VI" method="FP.Close"(reference=w404) -> (reference out=w403:refnum<vi>)  [unwired: 2 in, 2 out]
        n265 = invoke class="VI" method="Abort VI"(reference=w403) -> (error out=w402:errorcluster)  [unwired: 2 in, 2 out]
        n266 = invoke class="VI" method="Abort VI"(error in=w402) -> ()  [unwired: 2 in, 3 out]
      }
      event "Vision": Value Change {
        # "Enable/Disable Compression slider.\nHW USB is hard-coded into the camera"
        n267 = event-data() -> ("NewVal"=w410:u16)  [unwired: 1 in]
        n268 = Equal?(x=w410, y=u32 2 ("milliseconds to wait")) -> (x = y?=w408:bool)
        n269 = Select(t=T24."Disabled and Grayed Out" ("Disabled"), s=w408, f=T24."Enabled" ("Disabled")) -> (s? t:f=w405:T24)
        n270 = property on="Compression" class="Slide (strict)"("DisabledEnum"=w405) -> ()  [unwired: 2 in, 2 out]
      }
    }
  }
  n271 = while {
    tunnel: w41 -> [w413]
    i -> [w416]
    stop <- FALSE stop-if-true
    n272 = Wait (ms)(milliseconds to wait=u32 100) -> ()  [unwired: 1 out]
    n273 = case shown="\"Playback\"" "Rec Mode" {
      tunnel: w416 -> [_ _ w431]
      tunnel: [u32 2829099 ("Base Color") u32 11141120 ("Target Color") w420] -> w412
      frame "Stop", Default {
        # "Reset the color, extra updates don't cost much"
      }
      frame "Record" {
      }
      frame "Playback" {
        # "Playback"
        n274 = Quotient & Remainder(x=w431, y=u32 50 ("milliseconds to wait")) -> (x-y*floor(x/y)=w427:u32)  [unwired: 1 out]
        n275 = Divide(x=w427, y=u32 50 ("milliseconds to wait")) -> (x/y=w424:dbl)
        n276 = Multiply(x=6.283185307179586, y=w424) -> (x*y=w429:dbl)
        n277 = Sine(x=w429) -> (sin(x)=w428:dbl)
        n278 = Absolute Value(x=w428) -> (abs(x)=w421:dbl)
        n279 = call "Interpolate RGB Color.vi"("Proportion"=w421, "Target Color"=u32 30976, "Base Color"=u32 2829099) -> ("Result Color"=w420:u32)  [unwired: 8 in]
      }
    }
    n280 = property class="Pane"(reference=w413, "PaneColor"=w412) -> ()  [unwired: 1 in, 2 out]
  }
  n281 = TCP Create Listener(10:u16 1741 ("timeout ms (25000)")) -> (3:w5:refnum<k5>)  [unwired: 4 in, 2 out]
  n282 = while {
    tunnel: w5 -> [w433]
    stop <- FALSE stop-if-true
    n283 = TCP Wait On Listener(11:w433) -> (4:w432:refnum<k5>)  [unwired: 3 in, 4 out]
    n284 = local write "TCP"(w432) -> ()
  }
  n285 = property on="On/Off" class="Bool (strict)"("Visible"=w10) -> ()  [unwired: 2 in, 2 out]
  n286 = property on="Motor" class="Clust (strict)"("Visible"=w10) -> ()  [unwired: 2 in, 2 out]
  n287 = property on="Progress" class="Clust (strict)"("Visible"=w10) -> ()  [unwired: 2 in, 2 out]
  n288 = property on="Test Ring" class="Ring (strict)"("Visible"=w10) -> ()  [unwired: 2 in, 2 out]
  n289 = property on="Rev/Fwd" class="Clust (strict)"("Visible"=w10) -> ()  [unwired: 2 in, 2 out]
  n290 = local write "DB Camera Config"(w10) -> ()
  n291 = property on="Camera Settings" class="Clust (strict)"("Visible"=w10) -> ()  [unwired: 2 in, 2 out]
  n292 = global write "WPI_DashboardLogging Global.vi" "Recording"(w36) -> ()
  n293 = local write "Rec Mode"(w36) -> ()
